vi "setXmlParser.vi"(8 "error in (no error)":errorcluster, 10 "Tools.lvlib:xml.lvlib:XmlParser.lvclass":refnum<class "XmlParser.lvclass">, 11 "SettingsManager.lvclass in":refnum<class "SettingsManager.lvclass">) -> (0 "error out":errorcluster, 3 "SettingsManager.lvclass out":refnum<class "SettingsManager.lvclass">)   [LabVIEW 2011, in "Tools.lvlib" / "Settings.lvlib" / "SettingsManager.lvclass"]
uses:
  SettingsManager.lvclass
  XmlParser.lvclass
  SettingsManager.lvclass/SettingsManager.ctl
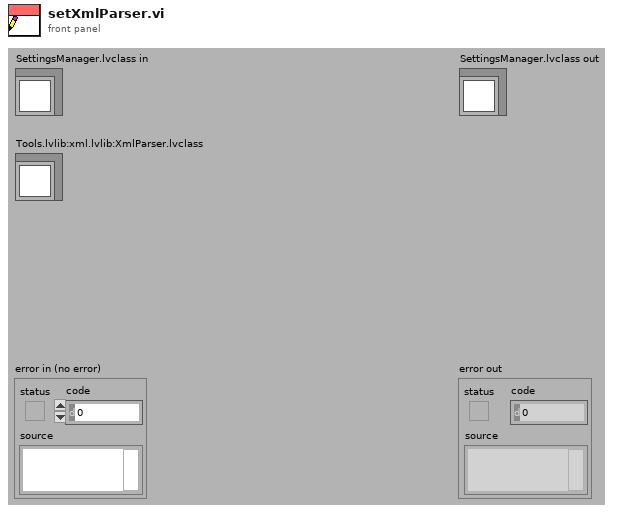
[diagram p1: front panel]
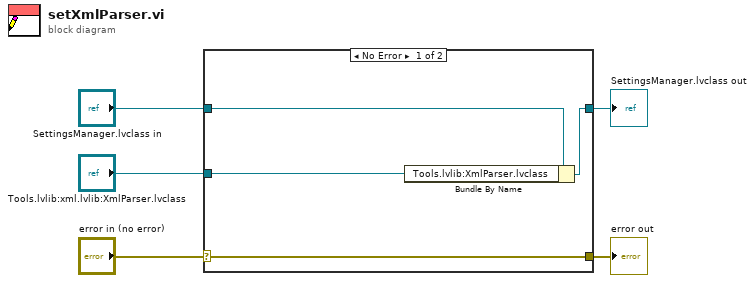
[diagram p0: block diagram]
diagram:
  n1 = case shown="No Error" "error in (no error)" {
    selector: "error in (no error)" -> [w9 w10]
    tunnel: [w9 w10] -> w4
    tunnel: [w7 w11] -> w2
    tunnel: "SettingsManager.lvclass in" -> [w8 w11]
    tunnel: "Tools.lvlib:xml.lvlib:XmlParser.lvclass" -> [w6 _]
    frame No Error {
      n2 = Bundle By Name(cluster=w8, "Tools.lvlib:XmlParser.lvclass"=w6) -> (w7:refnum<class "SettingsManager.lvclass">)
    }
    frame Error {
    }
  }
  "error out" <- w4
  "SettingsManager.lvclass out" <- w2
